vi "TAT_Start.vi"(8 "error In":errorcluster) -> (0 "error Out":errorcluster)   [LabVIEW 2017]
uses:
  Controls/Ass. Loop Control.ctl
  Controls/Torque Loop Control.ctl
  Controls/Data to DB.ctl
  <vilib>/NI/Modbus Library/API/master/Modbus Master.lvclass
  C:/Program Files (x86)/National Instruments/LabVIEW 2017/vi.lib/NI/Modbus Library/API/Modbus API.lvclass
  <vilib>/NI/Modbus Library/API/Wrapper/Create TCP Master.vi
  <vilib>/Instr/_visa.llb/VISA Configure Serial Port (Instr).vi
  <vilib>/addons/database/Connection.llb/DB Tools Open Connec (Path).vi
  <vilib>/addons/database/Auxilliary.llb/DB Tools Format Datetime String (Time Stamp).vi
  <vilib>/NI/Modbus Library/API/Wrapper/API Main.lvlib
  <vilib>/addons/database/NI_Database_API.lvlib
panel:
  out "Operator":bool
  out "Serial Number":string
  out "VARIENT":string
  out "USER":string
  in  "ASS-Alarms":bool
  in  "T-Alarms":bool
  in  "Stop Cycle":bool
  out "Torquing Result NOK":bool
  out "Torquing Result OK":bool
  out "FINAL BARCODE":string
  out "DAMPER BARCODE":string
  out "T-BODY BARCODE":string
  out "A-BODY BARCODE":string
  out "T-SPRING BARCODE":string
  out "OPERATION-A STATE":string
  out "GUN ENABLE":bool
  out "T-BIN-5":bool
  out "T-BIN-4":bool
  out "T-BIN-3":bool
  out "T-BIN-2":bool
  out "T-BIN-1":bool
  out "Ass Barcode OK":bool
  out "T BARCODE OK":bool
  out "TORQUE":string
  out "Torquing Cycle Reset":bool
  out "CYCLE START-T":bool
  out "Ass Cycle Reset":bool
  out "CYCLE START-A":bool
  out "OPERATION-T STATE":string
  out "PART SENSOR":bool
  out "PLC RUN":bool
  out "DATE/TIME":string
  out "BRACKET-2":bool
  out "BRACKET-1":bool
  out "A-SPRING BARCODE":string
  out "ASS. RESULT":string
  out "A-BIN-8":bool
  out "A-BIN-7":bool
  out "A-BIN-6":bool
  out "A-BIN-5":bool
  out "A-BIN-4":bool
  out "A-BIN-3":bool
  out "A-BIN-2":bool
  out "A-BIN-1":bool
  out "TORQUE RESULT":string
  in  "stop":bool
  # "STRUT PERIFERAL ASSEMBLY"
  # "TORQUING STATION"
  # "ASSEMBLY STATION"
  # "Nm"
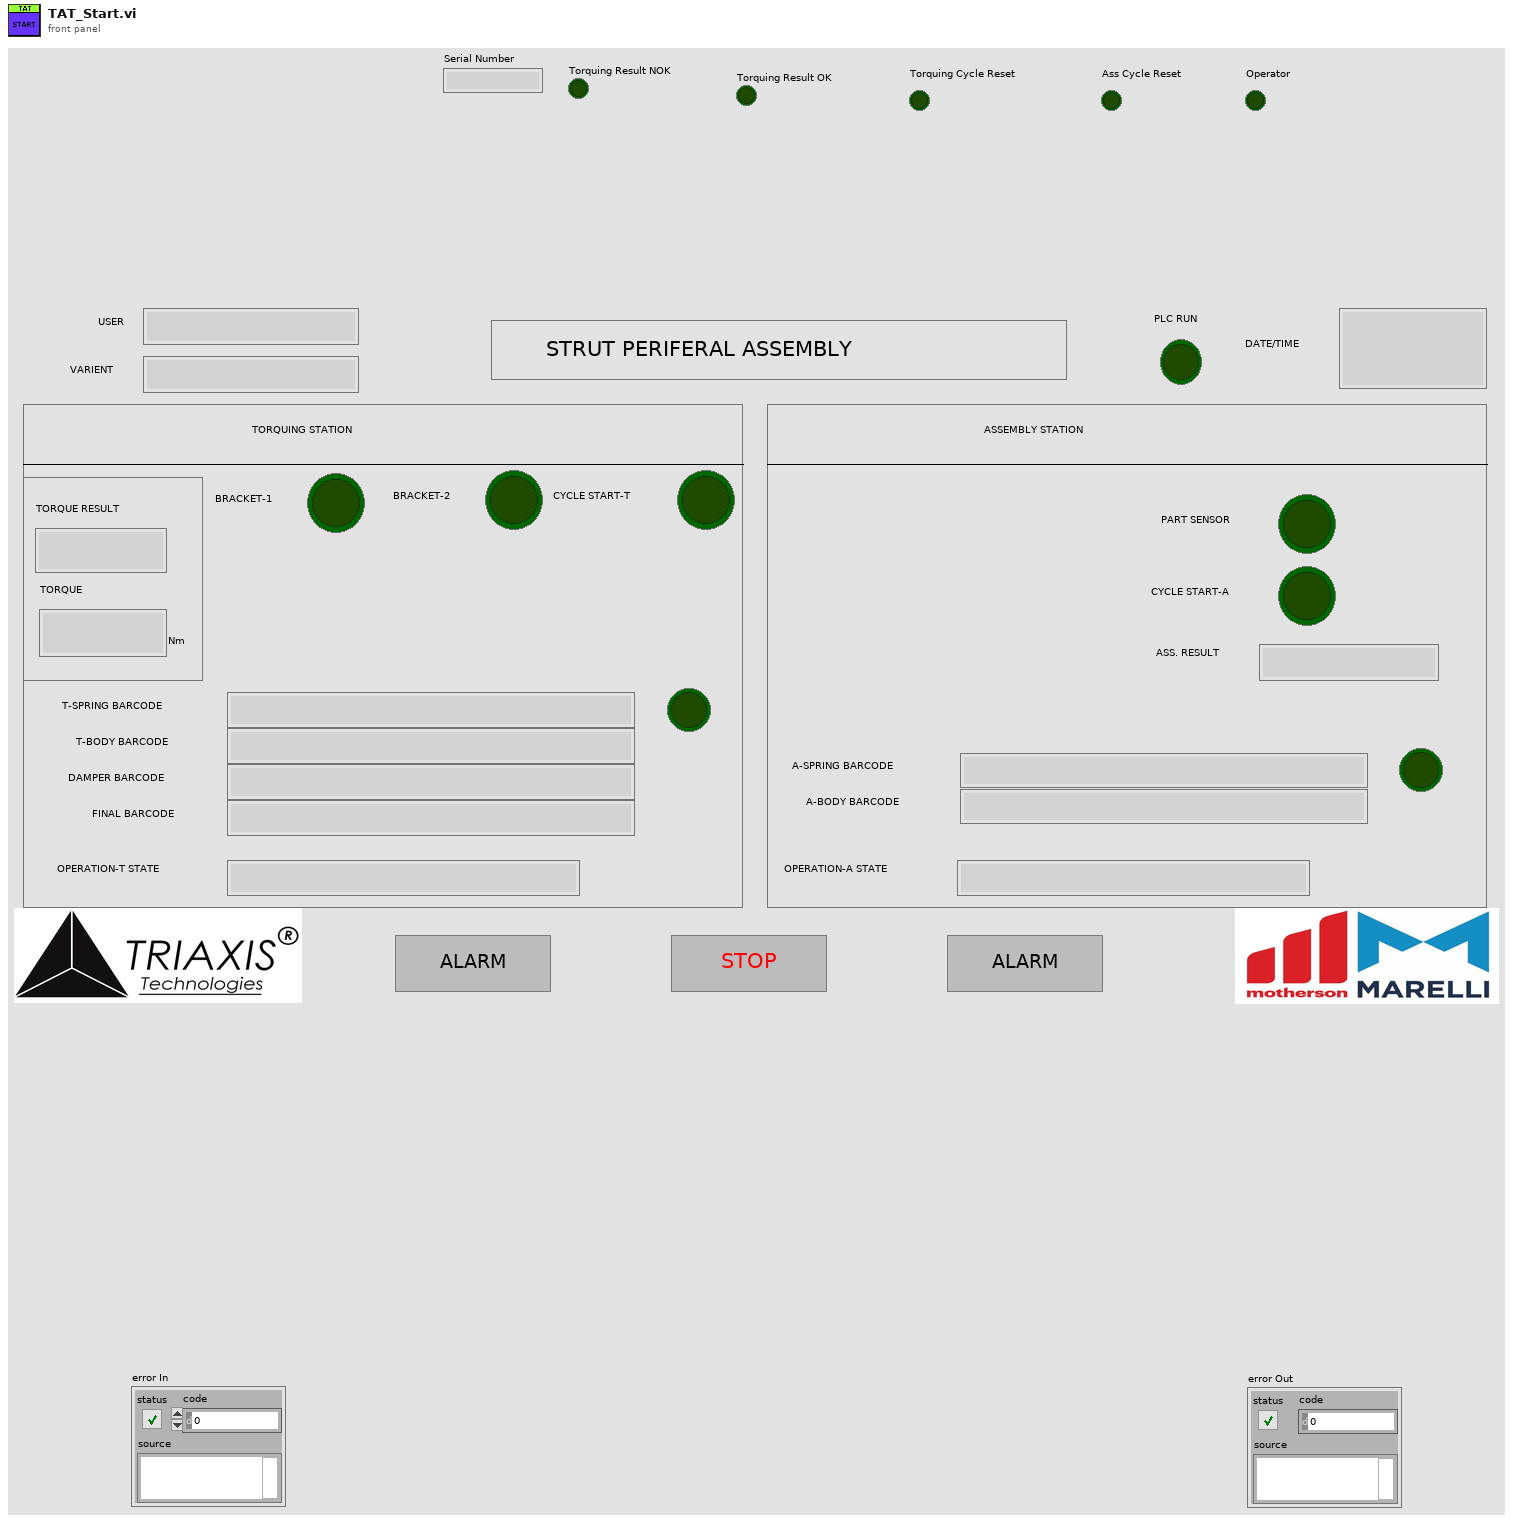
[diagram p1: front panel]
types:
  T1 = typedef "Torque Loop Control.ctl" = enum16{"Read T Spring Barcode", "Read T Body Barcode", "Read Damper Barcode", "T Start Cycle", "Wait for T Value", "Waiting For Result", "Waiting For Cycle End", "Print Final Barcode", "Update T Data", "T Cycle End"}
  T2 = typedef "Ass. Loop Control.ctl" = enum16{"Read Spring Barcode ", "Read Body Barcode", "Start Cycle", "Wait For Stop", "Cycle End", ""}
  T3 = enum32{"invalid app kind", "Development System", "Run Time System", "Student Edition", "Embedded LabVIEW", "Evaluation", "Custom"}
  T4 = typedef "NI_Database_API.lvlib/Conn ObjectReference.ctl" = refnum<k1>
  T5 = typedef "Recipe.ctl" = cluster{"Ass. Sensor Select":cluster{"Ass. Sensor Select":bool, "Camera-1 \nProg No.":u16, "Camera-2 \nProg No.":u16, "Gun \nProg No.":u16}, "Torque Sensor Select":cluster{"Torque Sensor-1":bool, "Torque Sensor-2":bool, "Torque Sensor-3":bool, "Torque Sensor-4":bool, "Torque Sensor-5":bool, "Torque Sensor-6":bool, "Torque Sensor-7":bool, "Torque Sensor-8":bool, "Torque Sensor-9":bool, "Torque Sensor-10":bool, "Torque Sensor-11":bool, "Torque Sensor-12":bool}, "Bin Seq. Select":cluster{"First Bin":u16, "Second Bin":u16, "Third Bin":u16, "Fourth Bin":u16, "Fifth Bin":u16, "Sixth Bin":u16, "Seventh Bin":u16, "Eighth Bin":u16, "Camera-1 Trig":u16, "Camera-2 Trig":u16}, "T-Bin Seq. Select":cluster{"First":u16, "Second":u16, "Third":u16, "Fourth":u16, "Fifth":u16, "Sixth":u16}, "Reference Barcode":cluster{"Spring Barcode":string, "Body Barcode":string, "14 Char of Barcode":string, "Final Barcode Length":string}, "Label Data":cluster{"Cust. Part No.":string, "TML Part No.":string, "Vendor Code":string, "Revision Level":string, "Part Description":string, "Vendor Name":string}}
  T6 = cluster{"First":u16, "Second":u16, "Third":u16, "Fourth":u16, "Fifth":u16, "Sixth":u16}
  T7 = cluster{"First Bin":u16, "Second Bin":u16, "Third Bin":u16, "Fourth Bin":u16, "Fifth Bin":u16, "Sixth Bin":u16, "Seventh Bin":u16, "Eighth Bin":u16, "Camera-1 Trig":u16, "Camera-2 Trig":u16}
  T8 = cluster{"Spring Barcode":string, "Body Barcode":string, "14 Char of Barcode":string, "Final Barcode Length":string}
  T9 = typedef "Data to DB.ctl" = cluster{"Date_Time":string, "Part_Name":string, "User_Code":string, "Damper_Barcode":string, "Serial_Number":string, "Assembly_Result":string, "Torque_value":string, "Torquing_Result":string, "Final_Barcode":string}
  T10 = typedef "Ass PLC Data Control.ctl" = cluster{"Cycle Start Ass":bool, "Bin-1":bool, "Bin-2":bool, "Bin-3":bool, "Bin-4":bool, "Bin-5":bool, "Bin-6":bool, "Bin-7":bool, "Bin-8":bool, "Ass Result OK":bool, "Ass Result NOK":bool, "PLC RUN":bool, "Part Sensor":bool, "Ass Cycle Reset":bool}
  T11 = typedef "Torque PLC Data Control.ctl" = cluster{"Cycle Start Torque":bool, "Bracket-1 Sensor":bool, "Bracket-2 Sensor":bool, "Torquing Result OK":bool, "Torquing Result NOK":bool, "Torquing Cycle Reset":bool, "T-BIN-1":bool, "T-BIN-2":bool, "T-BIN-3":bool, "T-BIN-4":bool, "T-BIN-5":bool, "T-BIN-6":bool}
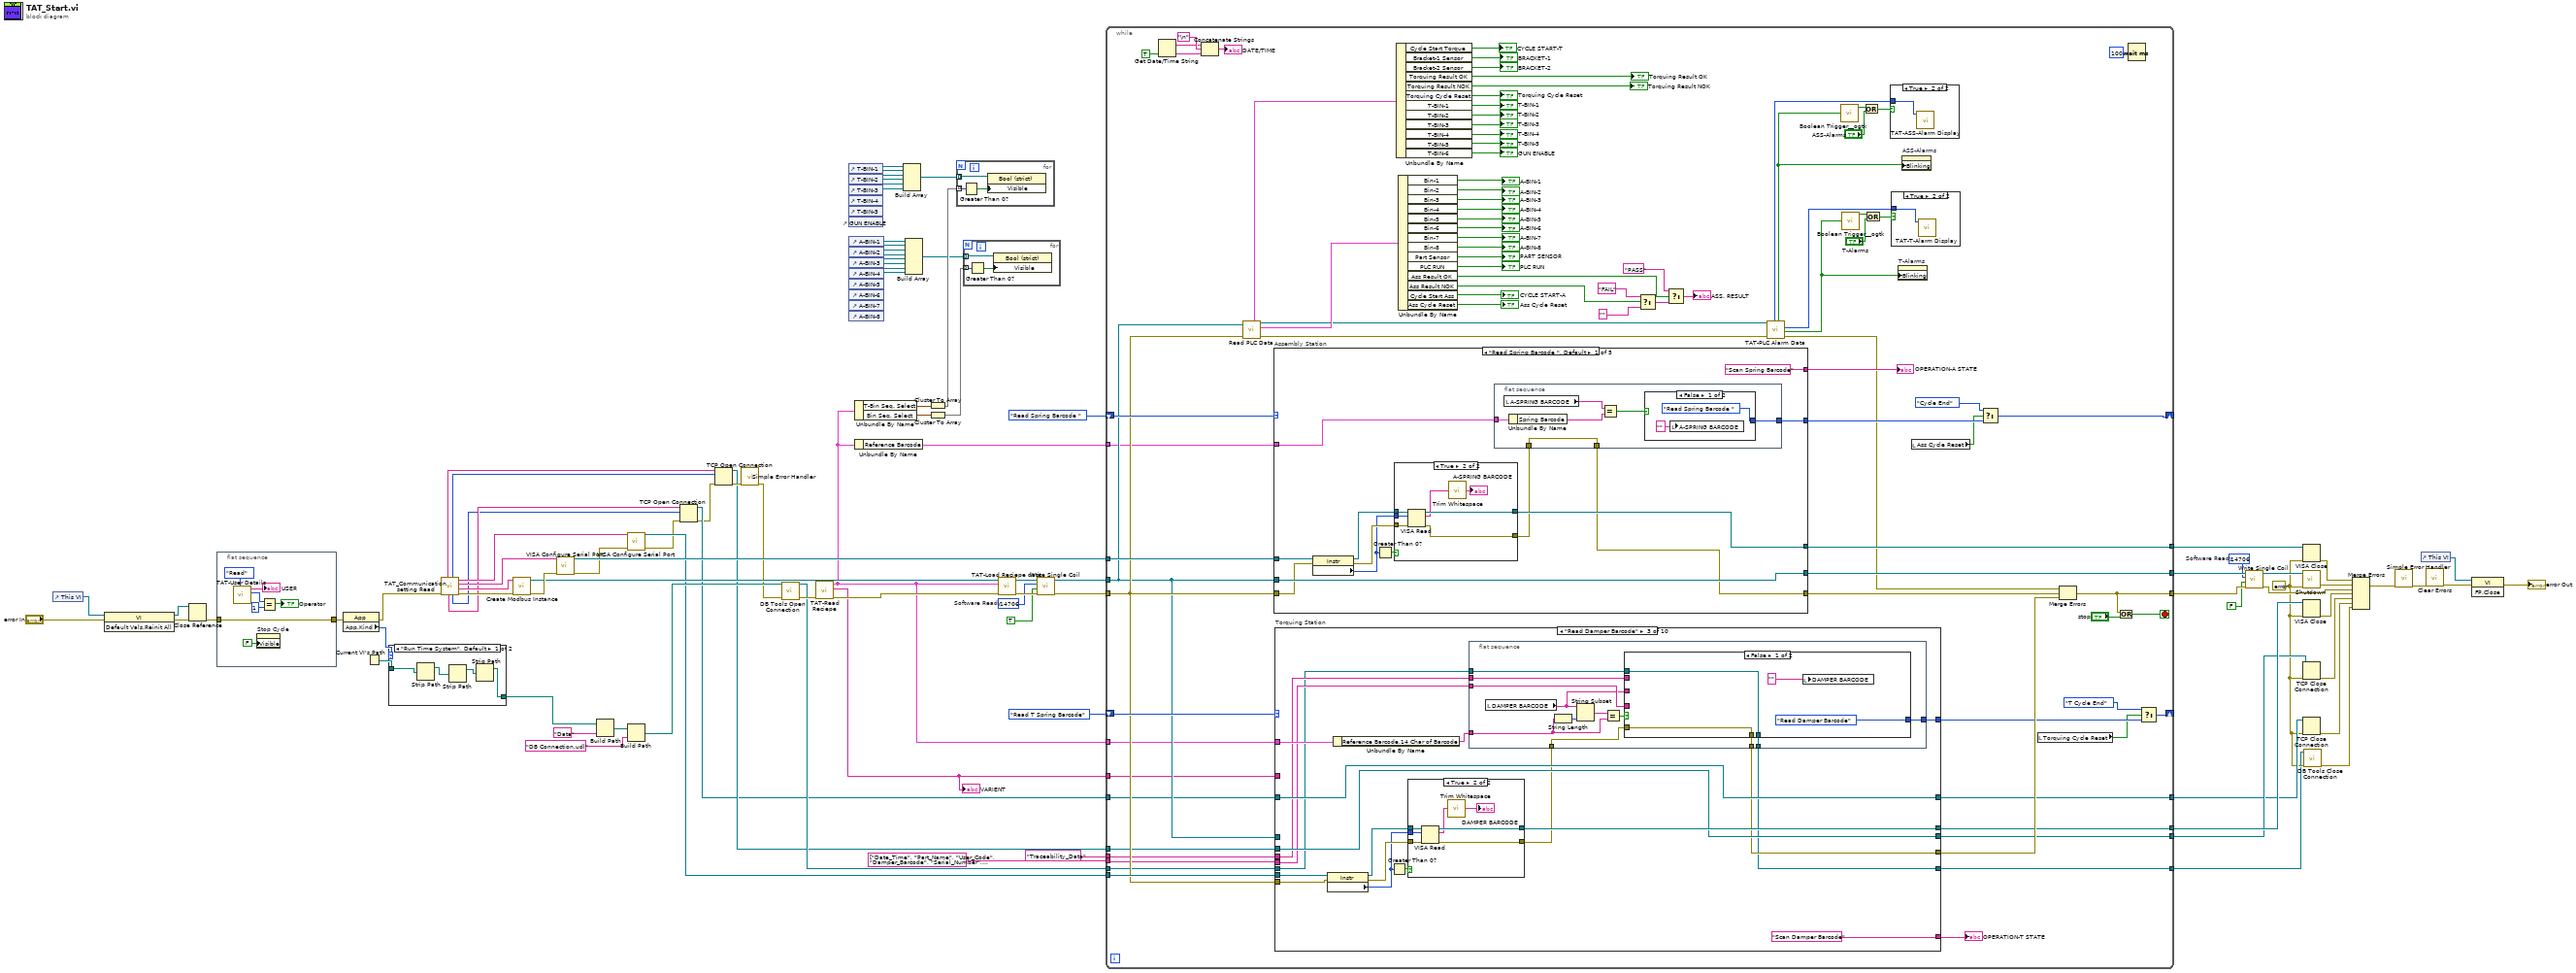
[diagram p0: block diagram]
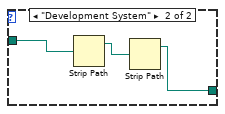
[diagram p2: hidden frame]
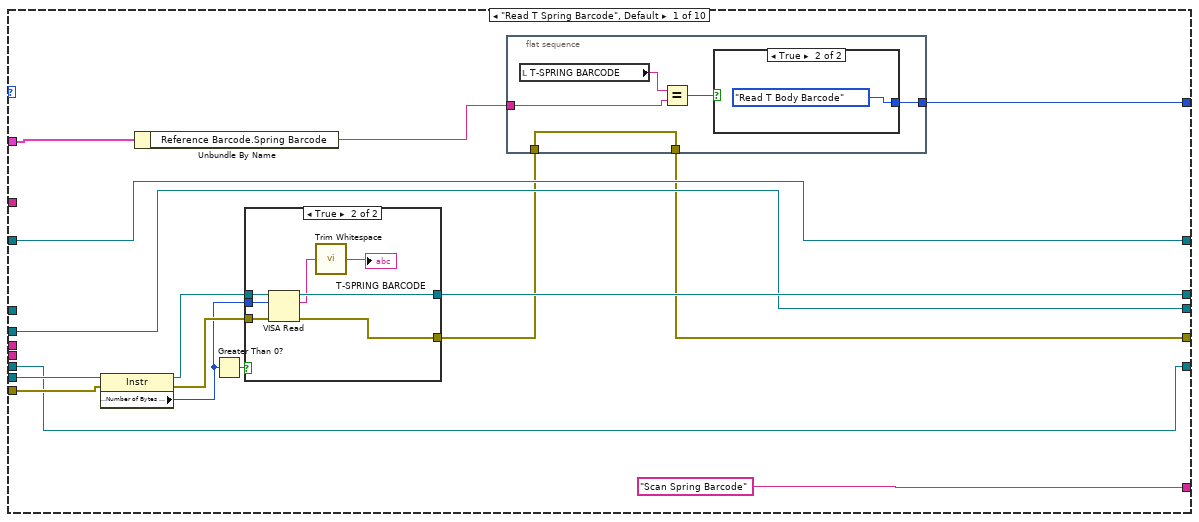
[diagram p5: hidden frame]
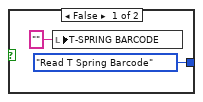
[diagram p6: hidden frame]
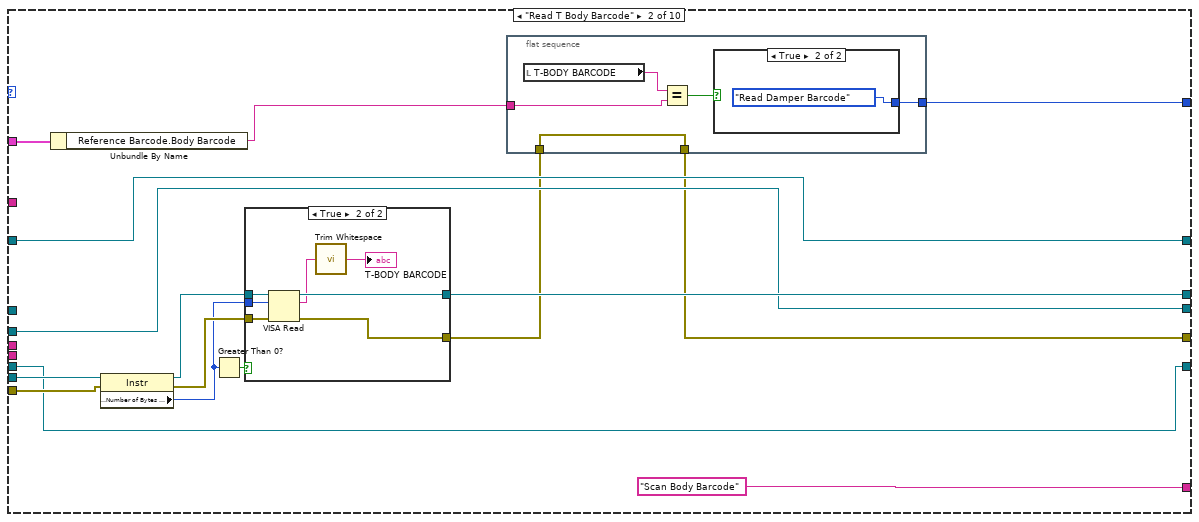
[diagram p8: hidden frame]
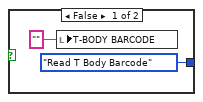
[diagram p9: hidden frame]
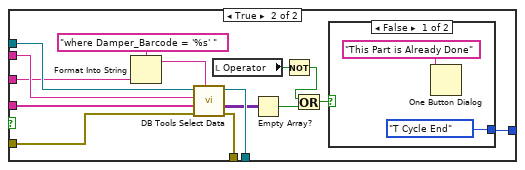
[diagram p11: hidden frame]
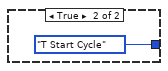
[diagram p12: hidden frame]
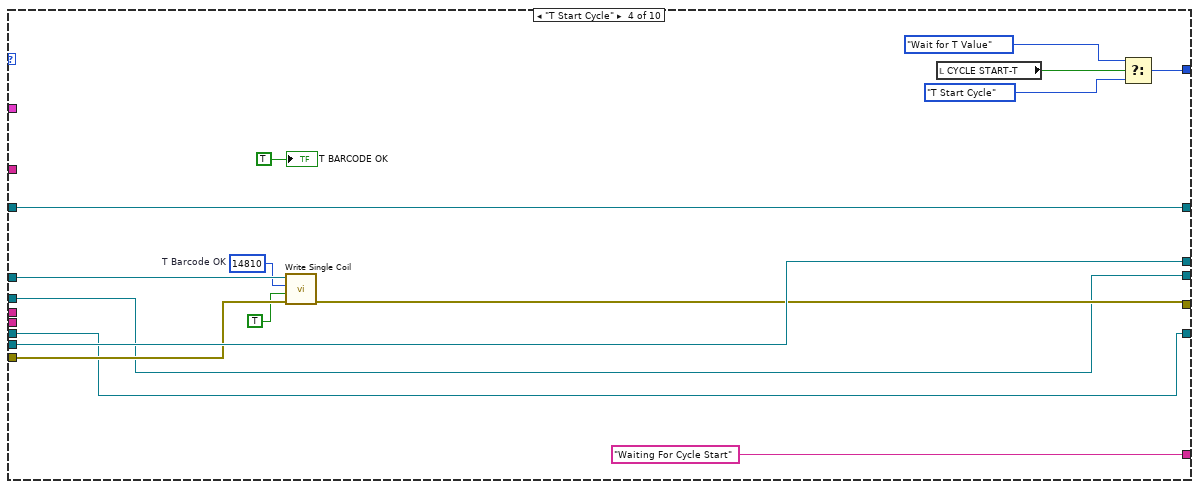
[diagram p14: hidden frame]
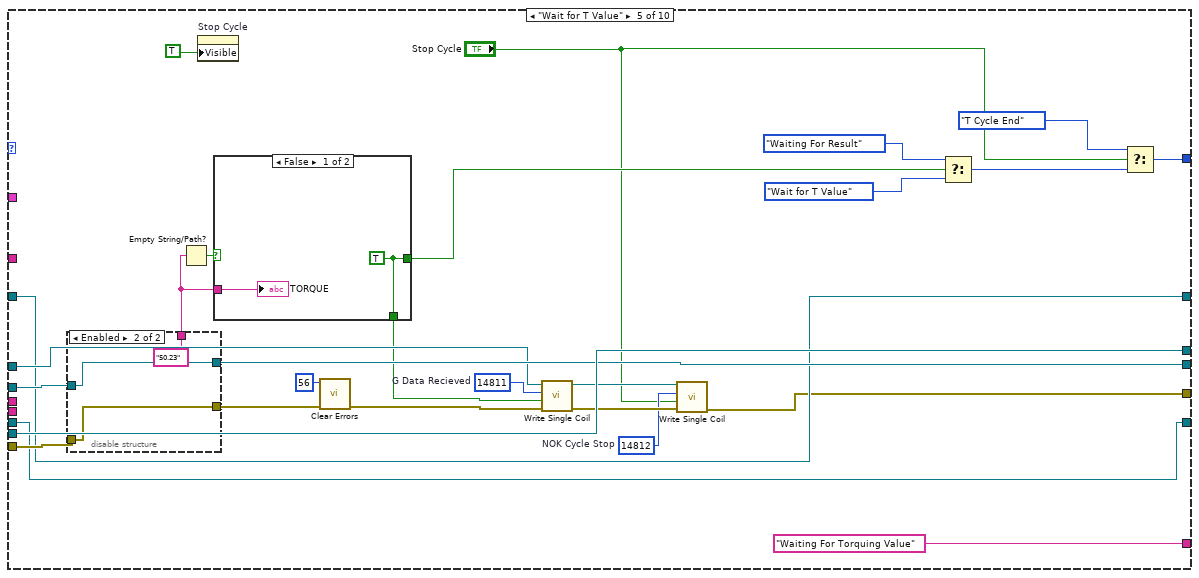
[diagram p15: hidden frame]
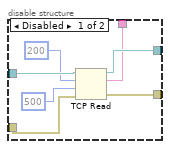
[diagram p16: hidden frame]
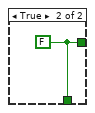
[diagram p17: hidden frame]
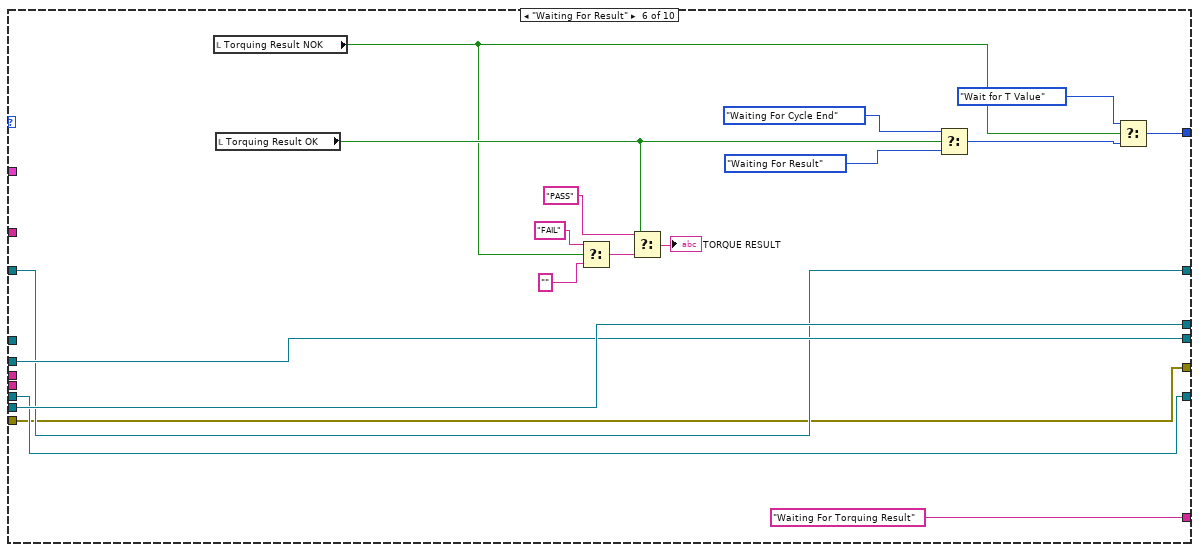
[diagram p18: hidden frame]
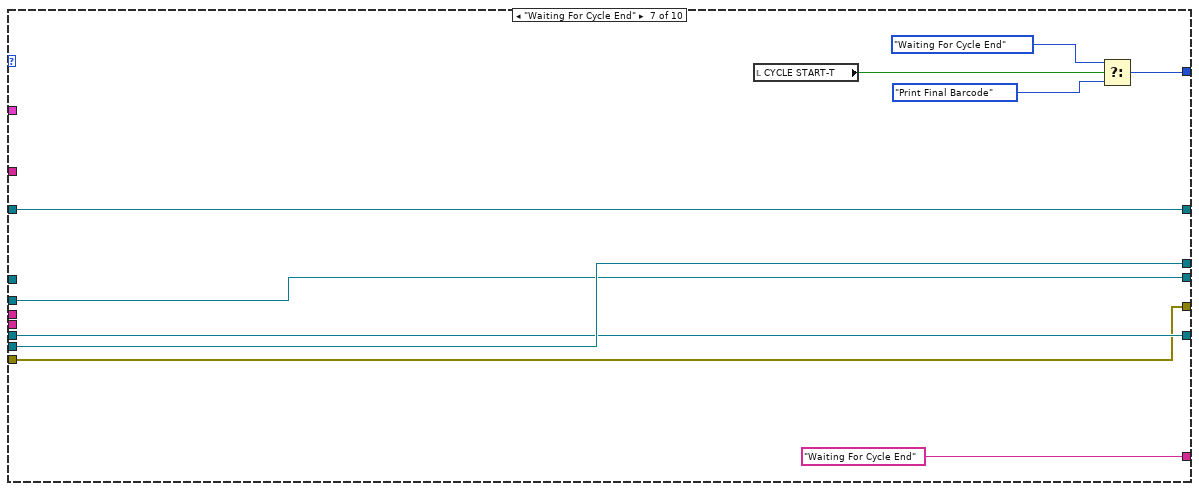
[diagram p19: hidden frame]
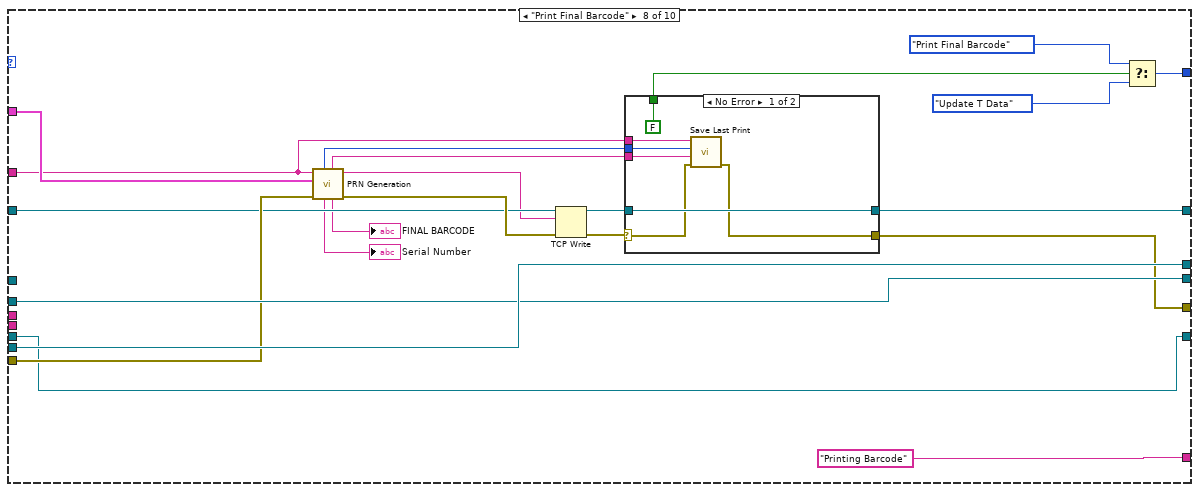
[diagram p20: hidden frame]
diagram:
  w41 = u16 14706  # Software Ready
  w69 = u16 14706  # Software Ready
  w12 = errorcluster {"status"=FALSE, "code"=0, "source"=""} ("error in")
  n1 = control-ref of="This VI"() -> (w39:refnum<vi>)
  n2 = invoke class="VI" method="Default Vals.Reinit All"(reference=w39, error in="error In") -> (reference out=w36:refnum<vi>, error out=w37:errorcluster)  [unwired: 1 in, 1 out]
  n3 = Close Reference(reference=w36, error in (no error)=w37) -> (error out=w4:errorcluster)
  n4 = flat-sequence {
    tunnel: [w99] -> w5
    tunnel: w4 -> [w99]
    frame #0 {
      n5 = call "TAT-User Details.vi"("Enum"=enum16{"Read", "Write"}."Read") -> ("Level Out"=w95:i32, "User Name Out"=→"USER":string)  [unwired: 9 in]
      n6 = property on="Stop Cycle" class="Bool"("Visible"=FALSE) -> ()  [unwired: 2 in, 2 out]
      n7 = Equal?(x=w95, y=1) -> (x = y?=→"Operator":bool)
    }
  }
  n8 = property class="App"(error in=w5) -> (error out=w48:errorcluster, "App.Kind"=w66:T3)  [unwired: 1 in, 1 out]
  n9 = Current VI's Path() -> (path=w67:path)
  n10 = case shown="\"Run Time System\", Default" w66 {
    tunnel: w67 -> [w101 w105]
    tunnel: [w100 w104] -> w49
    frame "Run Time System", Default {
      n11 = Strip Path(path=w101) -> (stripped path=w103:path)  [unwired: 1 out]
      n12 = Strip Path(path=w103) -> (stripped path=w102:path)  [unwired: 1 out]
      n13 = Strip Path(path=w102) -> (stripped path=w100:path)  [unwired: 1 out]
    }
    frame "Development System" {
      n14 = Strip Path(path=w105) -> (stripped path=w106:path)  [unwired: 1 out]
      n15 = Strip Path(path=w106) -> (stripped path=w104:path)  [unwired: 1 out]
    }
  }
  n16 = call "TAT_Communication setting Read.vi"("error in (no error)"=w48) -> ("error out"=w91:errorcluster, "PLC IP"=w88:string, "Ass Scanner Port"=w87:string, "Torque Scanner Port"=w85:string, "Printer Port"=w7:u32, "Screw Driver Port"=w9:u32, "Printer IP"=w8:string, "Screw Driver IP"=w82:string)  [unwired: 3 in]
  n17 = call-poly <vilib>:"Create Modbus Instance.vi"("error in"=w91, "address"=w88) -> ("error out"=w90:errorcluster, "TCP master instance"=w84:refnum<class "Modbus Master.lvclass">)  [unwired: 8 in]
  n18 = call-poly "VISA Configure Serial Port"("VISA resource name"=w87, "error in (no error)"=w90) -> ("VISA resource name out"=w89:refnum<visa-resource-name>, "error out"=w86:errorcluster)  [unwired: 12 in]
  n19 = Build Path(base path=w49, name or relative path="Data") -> (appended path=w50:path)
  n20 = call-poly "VISA Configure Serial Port"("VISA resource name"=w85, "error in (no error)"=w86) -> ("VISA resource name out"=w57:refnum<visa-resource-name>, "error out"=w15:errorcluster)  [unwired: 12 in]
  n21 = Build Path(base path=w50, name or relative path="DB Connection.udl") -> (appended path=w63:path)
  n22 = TCP Open Connection(address=w8, remote port or service name=w7, error in (no error)=w15) -> (connection ID=w47:refnum<k5>, error out=w14:errorcluster)  [unwired: 2 in]
  n23 = TCP Open Connection(address=w82, remote port or service name=w9, error in (no error)=w14) -> (connection ID=w54:refnum<k5>, error out=w62:errorcluster)  [unwired: 2 in]
  n24 = call <vilib>:"Simple Error Handler.vi"("error in (no error)"=w62) -> ("error out"=w6:errorcluster)  [unwired: 4 in, 4 out]
  n25 = call-poly <vilib>:"DB Tools Open Connection.vi"("error in (no error)"=w6, "connection information"=w63) -> ("error out"=w61:errorcluster, "connection reference"=w60:T4)  [unwired: 6 in]
  n26 = call "TAT-Read Reciepe.vi"("error in (no error)"=w61) -> ("error out"=w83:errorcluster, "Part Name"=w3:string, "Data To Load"=w2:T5)  [unwired: 8 in]
  "VARIENT" <- w3
  n27 = control-ref of="T-BIN-1"() -> (w27:refnum<vi>)
  n28 = control-ref of="T-BIN-2"() -> (w26:refnum<vi>)
  n29 = control-ref of="T-BIN-3"() -> (w25:refnum<vi>)
  n30 = control-ref of="T-BIN-4"() -> (w24:refnum<vi>)
  n31 = control-ref of="T-BIN-5"() -> (w23:refnum<vi>)
  n32 = control-ref of="GUN ENABLE"() -> (w22:refnum<vi>)
  n33 = control-ref of="A-BIN-1"() -> (w35:refnum<vi>)
  n34 = control-ref of="A-BIN-2"() -> (w34:refnum<vi>)
  n35 = control-ref of="A-BIN-3"() -> (w33:refnum<vi>)
  n36 = control-ref of="A-BIN-4"() -> (w32:refnum<vi>)
  n37 = control-ref of="A-BIN-5"() -> (w31:refnum<vi>)
  n38 = control-ref of="A-BIN-6"() -> (w30:refnum<vi>)
  n39 = control-ref of="A-BIN-7"() -> (w29:refnum<vi>)
  n40 = control-ref of="A-BIN-8"() -> (w28:refnum<vi>)
  n41 = Unbundle By Name(w2) -> ("T-Bin Seq. Select"=w17:T6, "Bin Seq. Select"=w16:T7)
  n42 = Unbundle By Name(w2) -> ("Reference Barcode"=w13:T8)
  n43 = Build Array(w27, w26, w25, w24, w23, w22) -> (w20:refnum<vi>[])
  n44 = Build Array(w35, w34, w33, w32, w31, w30, w29, w28) -> (w19:refnum<vi>[])
  n45 = Cluster To Array(cluster=w17) -> (array=w21:u16[])
  n46 = Cluster To Array(cluster=w16) -> (array=w18:u16[])
  n47 = for {
    tunnel: w21 -> [w109] mode=indexing
    tunnel: w20 -> [w108] mode=indexing
    n48 = Greater Than 0?(x=w109) -> (x > 0?=w107:bool)
    n49 = property class="Bool (strict)"(reference=w108, "Visible"=w107) -> ()  [unwired: 1 in, 2 out]
  }
  n50 = for {
    tunnel: w18 -> [w112] mode=indexing
    tunnel: w19 -> [w111] mode=indexing
    n51 = Greater Than 0?(x=w112) -> (x > 0?=w110:bool)
    n52 = property class="Bool (strict)"(reference=w111, "Visible"=w110) -> ()  [unwired: 1 in, 2 out]
  }
  n53 = call "TAT-Load Reciepe data.vi"("error in (no error)"=w83, "Ref Data"=w2, "Modbus Master in"=w84) -> ("error out"=w70:errorcluster, "Modbus Master out"=w73:refnum<class "Modbus Master.lvclass">)  [unwired: 7 in]
  n54 = call-dynamic "Write Single Coil.vi"("error in"=w70, "coil to write"=TRUE, "address"=w69, "Modbus master in"=w73) -> ("error out"=w71:errorcluster, "Modbus master out"=w72:refnum<class "Modbus Master.lvclass">)  [unwired: 6 in]
  n55 = while {
    tunnel: [w164] -> w43
    tunnel: w71 -> [w161]
    tunnel: w72 -> [w155]
    tunnel: w89 -> [w196]
    tunnel: w3 -> [w151]
    shift-right: [w137] -> _
    shift-left: Ass._Loop_Control."Read Spring Barcode " -> [w198]
    tunnel: [w195] -> w45
    tunnel: [w194] -> w81
    tunnel: w60 -> [w157]
    tunnel: "Traceability_Data" ("table") -> [w156]
    tunnel: string[] ["Date_Time", "Part_Name", "User_Code", "Damper_Barcode", "Serial_Number", "Assembly_Result", "Torque_Value", "Torquing_Result", "Final_Barcode"] -> [w140]
    shift-right: [w134] -> _
    shift-left: Torque_Loop_Control."Read T Spring Barcode" -> [w163]
    tunnel: w57 -> [w162]
    tunnel: [w159] -> w56
    tunnel: w54 -> [w154]
    tunnel: [w153] -> w51
    tunnel: w47 -> [w152]
    tunnel: [w150] -> w46
    tunnel: w13 -> [w141]
    tunnel: [w139] -> w11
    tunnel: w2 -> [w113]
    stop <- w166 stop-if-true
    n56 = Get Date/Time String(want seconds? (F)=TRUE) -> (date string=w115:string, time string=w114:string)  [unwired: 2 in]
    n57 = Concatenate Strings(w115, "\n", w114) -> (→"DATE/TIME":string)
    n58 = call "Read PLC Data.vi"("error in (no error)"=w161, "Modbus Master in"=w155) -> ("error out"=w130:errorcluster, "Ass PLC Data"=w178:T10, "Modbus Master out"=w128:refnum<class "Modbus Master.lvclass">, "Torque PLC Data"=w174:T11)  [unwired: 6 in]
    n59 = case "Assembly Station" shown="\"Read Spring Barcode \", Default" w198 {
      tunnel: w155 -> [w495 w526 w556 w564 w571]
      tunnel: w161 -> [w492 w523 w555 w563 w570]
      tunnel: w196 -> [w493 w524 w557 w565 w572]
      tunnel: [w494 w525 w549 w558 Ass._Loop_Control."Read Spring Barcode "] -> w138
      tunnel: [w485 w516 w553 w563 w570] -> w165
      tunnel: [w495 w526 w554 w564 w571] -> w195
      tunnel: [w487 w518 w557 w565 w572] -> w194
      tunnel: ["Scan Spring Barcode" "Scan Body Barcode" "Waiting for Start" "Waiting For Cycle End" "Cycle End"] -> w143
      tunnel: w141 -> [w483 w514 _ _ _]
      frame "Read Spring Barcode ", Default {
        n60 = property class="Instr"(reference=w493, error in=w492) -> (reference out=w491:refnum<visa-resource-name>, error out=w490:errorcluster, "Serial Settings:Number of Bytes at Serial Port"=w488:u32)
        n61 = Greater Than 0?(x=w488) -> (x > 0?=w489:bool)
        n62 = case shown="True" w489 {
          tunnel: w491 -> [w506 w513]
          tunnel: w490 -> [w505 w512]
          tunnel: w488 -> [_ w511]
          tunnel: [w506 w510] -> w487
          tunnel: [w505 w509] -> w484
          frame False {
          }
          frame True {
            n63 = VISA Read(VISA resource name=w513, byte count=w511, error in (no error)=w512) -> (VISA resource name out=w510:refnum<visa-resource-name>, read buffer=w507:string, error out=w509:errorcluster)  [unwired: 1 out]
            n64 = call <vilib>:"Trim Whitespace.vi"("string"=w507) -> ("trimmed string"=→"A-SPRING BARCODE":string)  [unwired: 1 in]
          }
        }
        n65 = flat-sequence {
          tunnel: [w496] -> w494
          tunnel: [w501] -> w485
          tunnel: w484 -> [w501]
          tunnel: w483 -> [w500]
          frame #0 {
            n66 = local read "A-SPRING BARCODE"() -> (w499:string)
            n67 = Unbundle By Name(w500) -> ("Spring Barcode"=w498:string)
            n68 = Equal?(x=w499, y=w498) -> (x = y?=w497:bool)
            n69 = case shown="False" w497 {
              tunnel: [Ass._Loop_Control."Read Spring Barcode " Ass._Loop_Control."Read Body Barcode"] -> w496
              frame False {
                n70 = local write "A-SPRING BARCODE"("" ("A-SPRING BARCODE")) -> ()
              }
              frame True {
              }
            }
          }
        }
      }
      frame "Read Body Barcode" {
        n71 = property class="Instr"(reference=w524, error in=w523) -> (reference out=w522:refnum<visa-resource-name>, error out=w521:errorcluster, "Serial Settings:Number of Bytes at Serial Port"=w519:u32)
        n72 = Greater Than 0?(x=w519) -> (x > 0?=w520:bool)
        n73 = case shown="True" w520 {
          tunnel: w522 -> [w537 w544]
          tunnel: w521 -> [w536 w543]
          tunnel: w519 -> [_ w542]
          tunnel: [w537 w541] -> w518
          tunnel: [w536 w540] -> w515
          frame False {
          }
          frame True {
            n74 = VISA Read(VISA resource name=w544, byte count=w542, error in (no error)=w543) -> (VISA resource name out=w541:refnum<visa-resource-name>, read buffer=w539:string, error out=w540:errorcluster)  [unwired: 1 out]
            n75 = call <vilib>:"Trim Whitespace.vi"("string"=w539) -> ("trimmed string"=→"A-BODY BARCODE":string)  [unwired: 1 in]
          }
        }
        n76 = flat-sequence {
          tunnel: [w527] -> w525
          tunnel: [w532] -> w516
          tunnel: w515 -> [w532]
          tunnel: w514 -> [w531]
          frame #0 {
            n77 = local read "A-BODY BARCODE"() -> (w530:string)
            n78 = Unbundle By Name(w531) -> ("Body Barcode"=w529:string)
            n79 = Equal?(x=w530, y=w529) -> (x = y?=w528:bool)
            n80 = case shown="True" w528 {
              tunnel: [Ass._Loop_Control."Read Body Barcode" Ass._Loop_Control."Start Cycle"] -> w527
              frame False {
                n81 = local write "A-BODY BARCODE"("" ("A-SPRING BARCODE")) -> ()
              }
              frame True {
              }
            }
          }
        }
      }
      frame "Start Cycle" {
        w552 = u16 14711  # Ass Barcode OK
        n82 = call-dynamic "Write Single Coil.vi"("error in"=w555, "coil to write"=TRUE, "address"=w552, "Modbus master in"=w556) -> ("error out"=w553:errorcluster, "Modbus master out"=w554:refnum<class "Modbus Master.lvclass">)  [unwired: 6 in]
        n83 = local read "CYCLE START-A"() -> (w548:bool)
        n84 = Select(t=Ass._Loop_Control."Wait For Stop", s=w548, f=Ass._Loop_Control."Start Cycle") -> (s? t:f=w549:T2)
        "Ass Barcode OK" <- TRUE ("Ass Barcode OK")
      }
      frame "Wait For Stop" {
        n85 = local read "CYCLE START-A"() -> (w560:bool)
        n86 = Select(t=Ass._Loop_Control."Wait For Stop", s=w560, f=Ass._Loop_Control."Cycle End") -> (s? t:f=w558:T2)
      }
      frame "Cycle End" {
        w566 = "" ("read buffer")
        n87 = local write "Ass Barcode OK"(FALSE ("Ass Barcode OK")) -> ()
        n88 = local write "A-SPRING BARCODE"(w566) -> ()
        n89 = local write "A-BODY BARCODE"(w566) -> ()
      }
    }
    "OPERATION-A STATE" <- w143
    n90 = case "Torquing Station" shown="\"Read Damper Barcode\"" w163 {
      tunnel: [w206 w239 w276 w335 w348 w393 w403 w421 Torque_Loop_Control."T Cycle End" Torque_Loop_Control."Read T Spring Barcode"] -> w133
      tunnel: w162 -> [w214 w247 w283 w344 w369 w400 w410 w434 w470 w481]
      tunnel: w161 -> [w213 w246 w282 w342 w367 w395 w405 w432 w472 w479]
      tunnel: [w205 w238 w270 w339 w352 w395 w405 w425 w466 w479] -> w160
      tunnel: [w211 w244 w280 w344 w369 w400 w410 w434 w470 w481] -> w159
      tunnel: w157 -> [w207 w240 w269 w330 w358 w396 w406 w427 w471 w475]
      tunnel: w156 -> [_ _ w272 _ _ _ _ _ w468 _]
      tunnel: w155 -> [_ _ _ w343 w364 _ _ _ _ _]
      tunnel: w154 -> [w210 w243 w279 w334 w368 w399 w409 w433 w469 w480]
      tunnel: [w210 w243 w279 w334 w366 w399 w409 w433 w469 w480] -> w153
      tunnel: w152 -> [w209 w242 w278 w333 w361 w398 w408 w430 w464 w478]
      tunnel: w151 -> [_ _ _ _ _ _ _ w416 w456 _]
      tunnel: [w209 w242 w278 w333 w361 w398 w408 w424 w464 w478] -> w150
      tunnel: ["Scan Spring Barcode" "Scan Body Barcode" "Scan Damper Barcode" "Waiting For Cycle Start" "Waiting For Torquing Value" "Waiting For Torquing Result" "Waiting For Cycle End" "Printing Barcode" "Save Data" "Cycle End"] -> w142
      tunnel: w140 -> [_ _ w271 _ _ _ _ _ w459 _]
      tunnel: [w207 w240 w268 w330 w358 w396 w406 w427 w458 w475] -> w139
      tunnel: w113 -> [w203 w236 w274 _ _ _ _ w418 _ _]
      frame "Read T Spring Barcode", Default {
        n91 = property class="Instr"(reference=w214, error in=w213) -> (reference out=w215:refnum<visa-resource-name>, error out=w216:errorcluster, "Serial Settings:Number of Bytes at Serial Port"=w212:u32)
        n92 = Unbundle By Name(w203) -> ("Reference Barcode.Spring Barcode"=w202:string)
        n93 = Greater Than 0?(x=w212) -> (x > 0?=w217:bool)
        n94 = case shown="True" w217 {
          tunnel: w215 -> [w227 w234]
          tunnel: w216 -> [w226 w233]
          tunnel: w212 -> [_ w232]
          tunnel: [w227 w231] -> w211
          tunnel: [w226 w230] -> w204
          frame False {
          }
          frame True {
            n95 = VISA Read(VISA resource name=w234, byte count=w232, error in (no error)=w233) -> (VISA resource name out=w231:refnum<visa-resource-name>, read buffer=w228:string, error out=w230:errorcluster)  [unwired: 1 out]
            n96 = call <vilib>:"Trim Whitespace.vi"("string"=w228) -> ("trimmed string"=→"T-SPRING BARCODE":string)  [unwired: 1 in]
          }
        }
        n97 = flat-sequence {
          tunnel: [w221] -> w206
          tunnel: [w219] -> w205
          tunnel: w204 -> [w219]
          tunnel: w202 -> [w218]
          frame #0 {
            n98 = local read "T-SPRING BARCODE"() -> (w222:string)
            n99 = Equal?(x=w222, y=w218) -> (x = y?=w220:bool)
            n100 = case shown="True" w220 {
              tunnel: [Torque_Loop_Control."Read T Spring Barcode" Torque_Loop_Control."Read T Body Barcode"] -> w221
              frame False {
                n101 = local write "T-SPRING BARCODE"("" ("T-SPRING BARCODE")) -> ()
              }
              frame True {
              }
            }
          }
        }
      }
      frame "Read T Body Barcode" {
        n102 = Unbundle By Name(w236) -> ("Reference Barcode.Body Barcode"=w235:string)
        n103 = property class="Instr"(reference=w247, error in=w246) -> (reference out=w248:refnum<visa-resource-name>, error out=w249:errorcluster, "Serial Settings:Number of Bytes at Serial Port"=w245:u32)
        n104 = Greater Than 0?(x=w245) -> (x > 0?=w250:bool)
        n105 = case shown="True" w250 {
          tunnel: w248 -> [w260 w267]
          tunnel: w249 -> [w259 w266]
          tunnel: w245 -> [_ w265]
          tunnel: [w260 w264] -> w244
          tunnel: [w259 w263] -> w237
          frame False {
          }
          frame True {
            n106 = VISA Read(VISA resource name=w267, byte count=w265, error in (no error)=w266) -> (VISA resource name out=w264:refnum<visa-resource-name>, read buffer=w262:string, error out=w263:errorcluster)  [unwired: 1 out]
            n107 = call <vilib>:"Trim Whitespace.vi"("string"=w262) -> ("trimmed string"=→"T-BODY BARCODE":string)  [unwired: 1 in]
          }
        }
        n108 = flat-sequence {
          tunnel: [w254] -> w239
          tunnel: [w252] -> w238
          tunnel: w237 -> [w252]
          tunnel: w235 -> [w251]
          frame #0 {
            n109 = local read "T-BODY BARCODE"() -> (w255:string)
            n110 = Equal?(x=w255, y=w251) -> (x = y?=w253:bool)
            n111 = case shown="True" w253 {
              tunnel: [Torque_Loop_Control."Read T Body Barcode" Torque_Loop_Control."Read Damper Barcode"] -> w254
              frame False {
                n112 = local write "T-BODY BARCODE"("" ("T-SPRING BARCODE")) -> ()
              }
              frame True {
              }
            }
          }
        }
      }
      frame "Read Damper Barcode" {
        n113 = property class="Instr"(reference=w283, error in=w282) -> (reference out=w284:refnum<visa-resource-name>, error out=w285:errorcluster, "Serial Settings:Number of Bytes at Serial Port"=w281:u32)
        n114 = Unbundle By Name(w274) -> ("Reference Barcode.14 Char of Barcode"=w273:string)
        n115 = Greater Than 0?(x=w281) -> (x > 0?=w286:bool)
        n116 = case shown="True" w286 {
          tunnel: w284 -> [w322 w329]
          tunnel: w285 -> [w321 w328]
          tunnel: w281 -> [_ w327]
          tunnel: [w322 w326] -> w280
          tunnel: [w321 w325] -> w275
          frame False {
          }
          frame True {
            n117 = VISA Read(VISA resource name=w329, byte count=w327, error in (no error)=w328) -> (VISA resource name out=w326:refnum<visa-resource-name>, read buffer=w324:string, error out=w325:errorcluster)  [unwired: 1 out]
            n118 = call <vilib>:"Trim Whitespace.vi"("string"=w324) -> ("trimmed string"=→"DAMPER BARCODE":string)  [unwired: 1 in]
          }
        }
        n119 = flat-sequence {
          tunnel: [w298] -> w276
          tunnel: w275 -> [w291]
          tunnel: w273 -> [w294]
          tunnel: w272 -> [w293]
          tunnel: w271 -> [w292]
          tunnel: [w290] -> w270
          tunnel: w269 -> [w289]
          tunnel: [w288] -> w268
          frame #0 {
            n120 = local read "DAMPER BARCODE"() -> (w287:string)
            n121 = String Length(string=w294) -> (length=w295:i32)
            n122 = String Subset(string=w287, length (rest)=w295) -> (substring=w296:string)  [unwired: 1 in]
            n123 = Equal?(x=w296, y=w294) -> (x = y?=w297:bool)
            n124 = case shown="False" w297 {
              tunnel: [Torque_Loop_Control."Read Damper Barcode" w306] -> w298
              tunnel: w293 -> [_ w317]
              tunnel: w292 -> [_ w316]
              tunnel: w291 -> [w300 w315]
              tunnel: [w300 w314] -> w290
              tunnel: w289 -> [w299 w313]
              tunnel: [w299 w312] -> w288
              tunnel: w287 -> [_ w310]
              frame False {
                n125 = local write "DAMPER BARCODE"("" ("T-SPRING BARCODE")) -> ()
              }
              frame True {
                n126 = Format Into String(format string="where Damper_Barcode = '%s' " ("condition"), w310) -> (resulting string=w309:string)  [unwired: 2 in, 1 out]
                n127 = call <vilib>:"DB Tools Select Data.vi"("condition"=w309, "error in (no error)"=w315, "columns"=w316, "table"=w317, "connection reference"=w313) -> ("error out"=w314:errorcluster, "data"=w308:variant[][], "connection reference out"=w312:T4)  [unwired: 1 in]
                n128 = local read "Operator"() -> (w303:bool)
                n129 = Empty Array?(array=w308) -> (empty?=w307:bool)
                n130 = Not(x=w303) -> (.not. x?=w304:bool)
                n131 = Or(x=w304, y=w307) -> (x .or. y?=w305:bool)
                n132 = case shown="False" w305 {
                  tunnel: [Torque_Loop_Control."T Cycle End" Torque_Loop_Control."T Start Cycle"] -> w306
                  frame False {
                    n133 = One Button Dialog(message="This Part is Already Done") -> ()  [unwired: 1 in, 1 out]
                  }
                  frame True {
                  }
                }
              }
            }
          }
        }
      }
      frame "T Start Cycle" {
        w341 = u16 14810  # T Barcode OK
        n134 = call-dynamic "Write Single Coil.vi"("error in"=w342, "coil to write"=TRUE, "address"=w341, "Modbus master in"=w343) -> ("error out"=w339:errorcluster)  [unwired: 6 in, 1 out]
        n135 = local read "CYCLE START-T"() -> (w336:bool)
        n136 = Select(t=Torque_Loop_Control."Wait for T Value", s=w336, f=Torque_Loop_Control."T Start Cycle") -> (s? t:f=w335:T1)
        "T BARCODE OK" <- TRUE
      }
      frame "Wait for T Value" {
        w350 = u16 14812  # NOK Cycle Stop
        w363 = u16 14811  # G Data Recieved
        n137 = disable-structure shown="Enabled" {
          disable-tunnel: w368 -> [w378 w381]
          disable-tunnel: w367 -> [w377 w380]
          disable-tunnel: [w376 w381] -> w366
          disable-tunnel: [w374 w380] -> w357
          disable-tunnel: [w373 "50.23" ("data out")] -> w355
          frame Disabled {
            n138 = TCP Read(connection ID=w378, bytes to read=200, error in (no error)=w377, 9:500 ("timeout ms (25000)")) -> (connection ID out=w376:refnum<k5>, data out=w373:string, error out=w374:errorcluster)  [unwired: 1 in]
          }
          frame Enabled {
          }
        }
        n139 = Empty String/Path?(string/path=w355) -> (empty?=w354:bool)
        n140 = property on="Stop Cycle" class="Bool"("Visible"=TRUE) -> ()  [unwired: 2 in, 2 out]
        n141 = case shown="False" w354 {
          tunnel: w355 -> [w383 _]
          tunnel: [w382 w384] -> w360
          tunnel: [w382 w384] -> w362
          frame False {
            w382 = TRUE
            "TORQUE" <- w383
          }
          frame True {
            w384 = FALSE
          }
        }
        n142 = call <vilib>:"Clear Errors.vi"("error in (no error)"=w357, "specific error code to clear (0: all)"=56) -> ("error out"=w365:errorcluster)  [unwired: 4 in, 1 out]
        n143 = call-dynamic "Write Single Coil.vi"("error in"=w365, "coil to write"=w362, "address"=w363, "Modbus master in"=w364) -> ("error out"=w353:errorcluster, "Modbus master out"=w351:refnum<class "Modbus Master.lvclass">)  [unwired: 6 in]
        n144 = call-dynamic "Write Single Coil.vi"("error in"=w353, "coil to write"="Stop Cycle", "address"=w350, "Modbus master in"=w351) -> ("error out"=w352:errorcluster)  [unwired: 6 in, 1 out]
        n145 = Select(t=Torque_Loop_Control."Waiting For Result", s=w360, f=Torque_Loop_Control."Wait for T Value") -> (s? t:f=w349:T1)
        n146 = Select(t=Torque_Loop_Control."T Cycle End", s="Stop Cycle", f=w349) -> (s? t:f=w348:T1)
      }
      frame "Waiting For Result" {
        n147 = local read "Torquing Result NOK"() -> (w385:bool)
        n148 = local read "Torquing Result OK"() -> (w386:bool)
        n149 = Select(t="FAIL", s=w385, f="") -> (s? t:f=w391:string)
        n150 = Select(t="PASS", s=w386, f=w391) -> (s? t:f=→"TORQUE RESULT":string)
        n151 = Select(t=Torque_Loop_Control."Waiting For Cycle End", s=w386, f=Torque_Loop_Control."Waiting For Result") -> (s? t:f=w394:T1)
        n152 = Select(t=Torque_Loop_Control."Wait for T Value", s=w385, f=w394) -> (s? t:f=w393:T1)
      }
      frame "Waiting For Cycle End" {
        n153 = local read "CYCLE START-T"() -> (w404:bool)
        n154 = Select(t=Torque_Loop_Control."Waiting For Cycle End", s=w404, f=Torque_Loop_Control."Print Final Barcode") -> (s? t:f=w403:T1)
      }
      frame "Print Final Barcode" {
        n155 = call "PRN Generation.vi"("error in (no error)"=w432, "Ref Data"=w418, "File Name"=w416) -> ("error out"=w431:errorcluster, "PRN to Print"=w429:string, "Barcode"=→"FINAL BARCODE":string, "Printing Date"=w414:string, "Serial Number"=→"Serial Number":string, "SN"=w415:u32)  [unwired: 3 in]
        n156 = TCP Write(connection ID=w430, data in=w429, error in (no error)=w431) -> (connection ID out=w423:refnum<k5>, error out=w426:errorcluster)  [unwired: 1 in, 1 out]
        n157 = case shown="No Error" w426 {
          selector: w426 -> [w439 _]
          tunnel: [w438 w446] -> w425
          tunnel: [w441 w445] -> w424
          tunnel: w423 -> [w441 _]
          tunnel: [FALSE TRUE] -> w419
          tunnel: w416 -> [w437 _]
          tunnel: w415 -> [w436 _]
          tunnel: w414 -> [w435 _]
          frame No Error {
            n158 = call "Save Last Print.vi"("error in (no error)"=w439, "Printing Date"=w435, "SN"=w436, "Part Name"=w437) -> ("error out"=w438:errorcluster)  [unwired: 7 in]
          }
          frame Error {
            n159 = call "TAT_Communication setting Read.vi"("error in (no error)"=errorcluster {"status"=FALSE, "code"=0, "source"=""}) -> ("error out"=w447:errorcluster, "Printer Port"=w443:u32, "Printer IP"=w444:string)  [unwired: 3 in, 5 out]
            n160 = TCP Open Connection(address=w444, remote port or service name=w443, error in (no error)=w447) -> (connection ID=w445:refnum<k5>, error out=w446:errorcluster)  [unwired: 2 in]
          }
        }
        n161 = Select(t=Torque_Loop_Control."Print Final Barcode", s=w419, f=Torque_Loop_Control."Update T Data") -> (s? t:f=w421:T1)
      }
      frame "Update T Data" {
        n162 = local read "DAMPER BARCODE"() -> (w454:string)
        n163 = local read "TORQUE"() -> (w452:string)
        n164 = local read "FINAL BARCODE"() -> (w450:string)
        n165 = call "TAT-User Details.vi"("Enum"=enum16{"Read", "Write"}."Read") -> ("User Name Out"=w455:string)  [unwired: 9 in, 1 out]
        n166 = call-poly <vilib>:"DB Tools Format Datetime String.vi"() -> ("date/time string"=w457:string)  [unwired: 1 in]
        n167 = local read "Serial Number"() -> (w449:string)
        n168 = Bundle By Name(cluster=T9 {"Date_Time"="", "Part_Name"="", "User_Code"="", "Damper_Barcode"="", "Serial_Number"="", "Assembly_Result"="", "Torque_value"="", "Torquing_Result"="", "Final_Barcode"=""}, "Date_Time"=w457, "Part_Name"=w456, "User_Code"=w455, "Damper_Barcode"=w454, "Serial_Number"=w449, "Assembly_Result"="OK", "Torque_value"=w452, "Torquing_Result"="OK", "Final_Barcode"=w450) -> (w461:T9)
        n169 = To Variant(anything=w461) -> (Variant=w467:variant)
        n170 = call <vilib>:"DB Tools Insert Data.vi"("data"=w467, "error in (no error)"=w472, "columns"=w459, "table"=w468, "connection reference"=w471) -> ("error out"=w466:errorcluster, "connection reference out"=w458:T4)  [unwired: 5 in]
      }
      frame "T Cycle End" {
        w473 = "" ("read buffer")
        n171 = property on="Stop Cycle" class="Bool"("Visible"=FALSE) -> ()  [unwired: 2 in, 2 out]
        n172 = local write "T BARCODE OK"(FALSE ("T Barcode OK")) -> ()
        n173 = local write "T-SPRING BARCODE"(w473) -> ()
        n174 = local write "T-BODY BARCODE"(w473) -> ()
        n175 = local write "DAMPER BARCODE"(w473) -> ()
      }
    }
    "OPERATION-T STATE" <- w142
    n176 = Unbundle By Name(w174) -> ("Cycle Start Torque"=→"CYCLE START-T":bool, "Bracket-1 Sensor"=→"BRACKET-1":bool, "Bracket-2 Sensor"=→"BRACKET-2":bool, "Torquing Result OK"=→"Torquing Result OK":bool, "Torquing Result NOK"=→"Torquing Result NOK":bool, "Torquing Cycle Reset"=→"Torquing Cycle Reset":bool, "T-BIN-1"=→"T-BIN-1":bool, "T-BIN-2"=→"T-BIN-2":bool, "T-BIN-3"=→"T-BIN-3":bool, "T-BIN-4"=→"T-BIN-4":bool, "T-BIN-5"=→"T-BIN-5":bool, "T-BIN-6"=→"GUN ENABLE":bool)
    n177 = Unbundle By Name(w178) -> ("Bin-1"=→"A-BIN-1":bool, "Bin-2"=→"A-BIN-2":bool, "Bin-3"=→"A-BIN-3":bool, "Bin-4"=→"A-BIN-4":bool, "Bin-5"=→"A-BIN-5":bool, "Bin-6"=→"A-BIN-6":bool, "Bin-7"=→"A-BIN-7":bool, "Bin-8"=→"A-BIN-8":bool, "Part Sensor"=→"PART SENSOR":bool, "PLC RUN"=→"PLC RUN":bool, "Ass Result OK"=w190:bool, "Ass Result NOK"=w191:bool, "Cycle Start Ass"=→"CYCLE START-A":bool, "Ass Cycle Reset"=→"Ass Cycle Reset":bool)
    n178 = Select(t="FAIL", s=w191, f="") -> (s? t:f=w189:string)
    n179 = Select(t="PASS", s=w190, f=w189) -> (s? t:f=→"ASS. RESULT":string)
    n180 = call "TAT-PLC Alarm Data.vi"("error in (no error)"=w130, "Modbus instance in"=w128) -> ("error out"=w129:errorcluster, "Alarm Enable-2"=w118:bool, "T - Alarm"=w120:u16[], "Alarm Enable-1"=w119:bool, "Ass Alarm"=w124:u16[])  [unwired: 4 in, 1 out]
    n181 = call <userlib>:"Boolean Trigger__ogtk.vi"("Boolean Input"=w119) -> ("Rising Edge"=w127:bool)  [unwired: 1 in, 1 out]
    n182 = call <userlib>:"Boolean Trigger__ogtk.vi"("Boolean Input"=w118) -> ("Rising Edge"=w123:bool)  [unwired: 1 in, 1 out]
    n183 = Or(x=w127, y="ASS-Alarms") -> (x .or. y?=w126:bool)
    n184 = Or(x=w123, y="T-Alarms") -> (x .or. y?=w121:bool)
    n185 = case shown="True" w126 {
      tunnel: w124 -> [_ w201]
      frame False {
      }
      frame True {
        n186 = call "TAT-ASS-Alarm Display.vi"("Ass Alarm"=w201) -> ()  [unwired: 11 in]
      }
    }
    n187 = case shown="True" w121 {
      tunnel: w120 -> [_ w200]
      frame False {
      }
      frame True {
        n188 = call "TAT-T-Alarm Display.vi"("T-Alarm"=w200) -> ()  [unwired: 11 in]
      }
    }
    n189 = property on="T-Alarms" class="Bool"("Blinking"=w118) -> ()  [unwired: 2 in, 2 out]
    n190 = property on="ASS-Alarms" class="Bool"("Blinking"=w119) -> ()  [unwired: 2 in, 2 out]
    n191 = local read "Ass Cycle Reset"() -> (w136:bool)
    n192 = Select(t=Ass._Loop_Control."Cycle End", s=w136, f=w138) -> (s? t:f=w137:T2)
    n193 = local read "Torquing Cycle Reset"() -> (w131:bool)
    n194 = Merge Errors(w129, w165, w160) -> (w164:errorcluster)
    n195 = Or(x=w164, y="stop") -> (x .or. y?=w166:bool)
    n196 = Wait (ms)(milliseconds to wait=u32 100) -> ()  [unwired: 1 out]
    n197 = Select(t=Torque_Loop_Control."T Cycle End", s=w131, f=w133) -> (s? t:f=w134:T1)
  }
  n198 = call-dynamic "Write Single Coil.vi"("error in"=w43, "coil to write"=FALSE, "address"=w41, "Modbus master in"=w45) -> ("error out"=w42:errorcluster, "Modbus master out"=w44:refnum<class "Modbus Master.lvclass">)  [unwired: 6 in]
  n199 = call-dynamic "Shutdown.vi"("error in"=w12, "Modbus master in"=w44) -> ("error out"=w79:errorcluster)  [unwired: 9 in]
  n200 = VISA Close(VISA resource name=w56, error in (no error)=w12) -> (error out=w55:errorcluster)
  n201 = VISA Close(VISA resource name=w81, error in (no error)=w12) -> (error out=w80:errorcluster)
  n202 = TCP Close Connection(connection ID=w51, error in (no error)=w12) -> (error out=w53:errorcluster)  [unwired: 1 in, 1 out]
  n203 = TCP Close Connection(connection ID=w46, error in (no error)=w12) -> (error out=w52:errorcluster)  [unwired: 1 in, 1 out]
  n204 = call <vilib>:"DB Tools Close Connection.vi"("error in (no error)"=w12, "connection reference"=w11) -> ("error out"=w10:errorcluster)  [unwired: 5 in]
  n205 = Merge Errors(w80, w79, w42, w55, w53, w52, w10) -> (w78:errorcluster)
  n206 = call <vilib>:"Simple Error Handler.vi"("error in (no error)"=w78) -> ("error out"=w77:errorcluster)  [unwired: 4 in, 4 out]
  n207 = control-ref of="This VI"() -> (w75:refnum<vi>)
  n208 = call <vilib>:"Clear Errors.vi"("error in (no error)"=w77) -> ("error out"=w76:errorcluster)  [unwired: 5 in, 1 out]
  n209 = invoke class="VI" method="FP.Close"(reference=w75, error in=w76) -> (error out=→"error Out":errorcluster)  [unwired: 1 in, 2 out]
